vi "Read CSV File.vi"(11 "file path (dialog if empty)":path) -> (3 "signals":bool[][](array[boolean]))   [LabVIEW 2013]
uses:
  <vilib>/Utility/file.llb/Read From Spreadsheet File (I64).vi
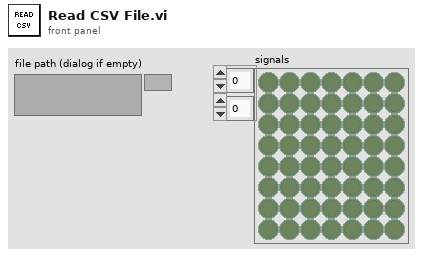
[diagram p1: front panel]
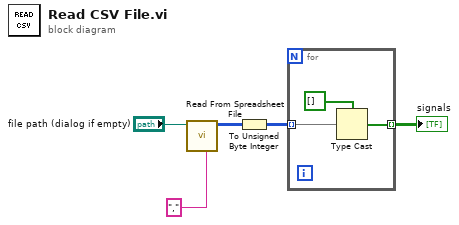
[diagram p0: block diagram]
diagram:
  n1 = call-poly <vilib>:"Read From Spreadsheet File.vi"("delimiter (\\t)"="," ("delimiter (\\t)"), "file path (dialog if empty)"="file path (dialog if empty)") -> ("all rows"=w4:i64[][])  [unwired: 5 in, 4 out]
  n2 = To Unsigned Byte Integer(number=w4) -> (unsigned 8bit integer=w3:u8[][])
  n3 = for {
    tunnel: w3 -> [w8] mode=indexing
    tunnel: [w6] -> w2 mode=indexing
    n4 = Type Cast(type=bool[] [], x=w8) -> (*(type *) &x=w6:bool[])
  }
  "signals" <- w2
